vi "Get Run URL.vi"(8 "error in (no error)":errorcluster, 10 "Run ID":string, 11 "Sift Client in":refnum<class "Sift Client.lvclass">) -> (0 "error out":errorcluster, 2 "URL":string, 3 "Sift Client out":refnum<class "Sift Client.lvclass">)   [LabVIEW 2024, in "Sift Client.lvlib" / "Sift Client.lvclass"]
doc: "Get the URL for a given Run ID."
uses:
  Sift Client.lvclass
  Sift Client.lvclass/Sift Client.ctl
  <vilib>/regexp/Match Regular Expression.xnode
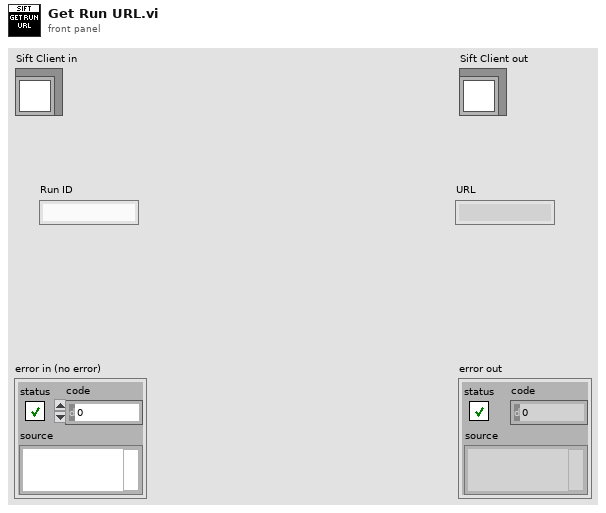
[diagram p1: front panel]
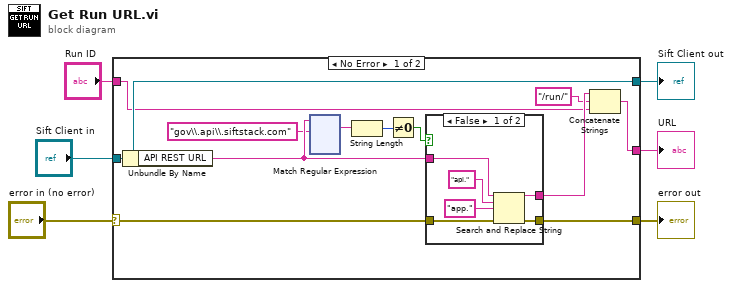
[diagram p0: block diagram]
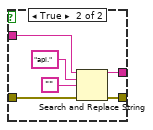
[diagram p2: hidden frame]
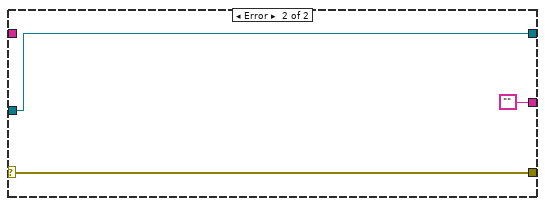
[diagram p3: hidden frame]
diagram:
  n1 = case shown="No Error" "error in (no error)" {
    selector: "error in (no error)" -> [w13 w150]
    tunnel: [w12 w150] -> w5
    tunnel: [w18 w149] -> w3
    tunnel: "Sift Client in" -> [w18 w149]
    tunnel: "Run ID" -> [w15 _]
    tunnel: [w14 ""] -> w1
    frame No Error {
      n2 = Unbundle By Name(w18) -> ("API REST URL"=w11:string)
      n3 = xnode "Match Regular Expression"("input string"=w11, "regular expression"="gov\\.api\\.siftstack.com") -> ("whole match"=w9:string)  [unwired: 4 in, 4 out]
      n4 = String Length(string=w9) -> (length=w8:i32)
      n5 = Not Equal To 0?(x=w8) -> (x != 0?=w7:bool)
      n6 = case shown="False" w7 {
        tunnel: w11 -> [w141 w146]
        tunnel: [w138 w144] -> w17
        tunnel: w13 -> [w137 w143]
        tunnel: [w136 w142] -> w12
        frame False {
          n7 = Search and Replace String(input string=w141, search string="api.", replace string="app." ("replace string (\"\")"), error in=w137) -> (result string=w138:string, error out=w136:errorcluster)  [unwired: 4 in, 2 out]
        }
        frame True {
          n8 = Search and Replace String(input string=w146, search string="api.", replace string="", error in=w143) -> (result string=w144:string, error out=w142:errorcluster)  [unwired: 4 in, 2 out]
        }
      }
      n9 = Concatenate Strings(w17, "/run/" ("string"), w15) -> (w14:string)
    }
    frame Error {
    }
  }
  "error out" <- w5
  "Sift Client out" <- w3
  "URL" <- w1
